vi "EINDE.vi"() -> ()   [LabVIEW 2018]
uses:
  Kleuren- en afstandsensor/FSM States.ctl
  FSM States Project TOTAAL.ctl
panel:
  out "Genoeg blokjes?":bool
  out "Initial State":T1=enum."MOVE DOWNWARDS"
  out "Tussentijd":i32
  out "Timer2":i32
  out "The End":bool
  in  "stop 3":bool
  in  "ON/OFF Grijper":bool
  in  "stop":bool
  in  "Aantal Witte blokjes":dbl
  in  "Aantal rode blokjes":dbl
  in  "Aantal Zwarte blokjes":dbl
  in  "LED aansturen":bool[](array[boolean])
  out "Current State":T1
  out "Motor":bool[](array[boolean])
  out "State to recover from":T1=enum."Stilstaan"
  in  "EMERGENCY":bool
  in  "Teller wit":dbl
  in  "Teller Rood":dbl
  in  "Teller zwart":dbl
  out "Wit":bool
  out "Zwart":bool
  out "Rood":bool
  in  "Kleurmaken":bool
  out "Kleuren veranderen":T2
  out "Analoge in":dbl[](array[numeric]) format="%0.2f"
  out "Afstand":bool
  # "INPUT"
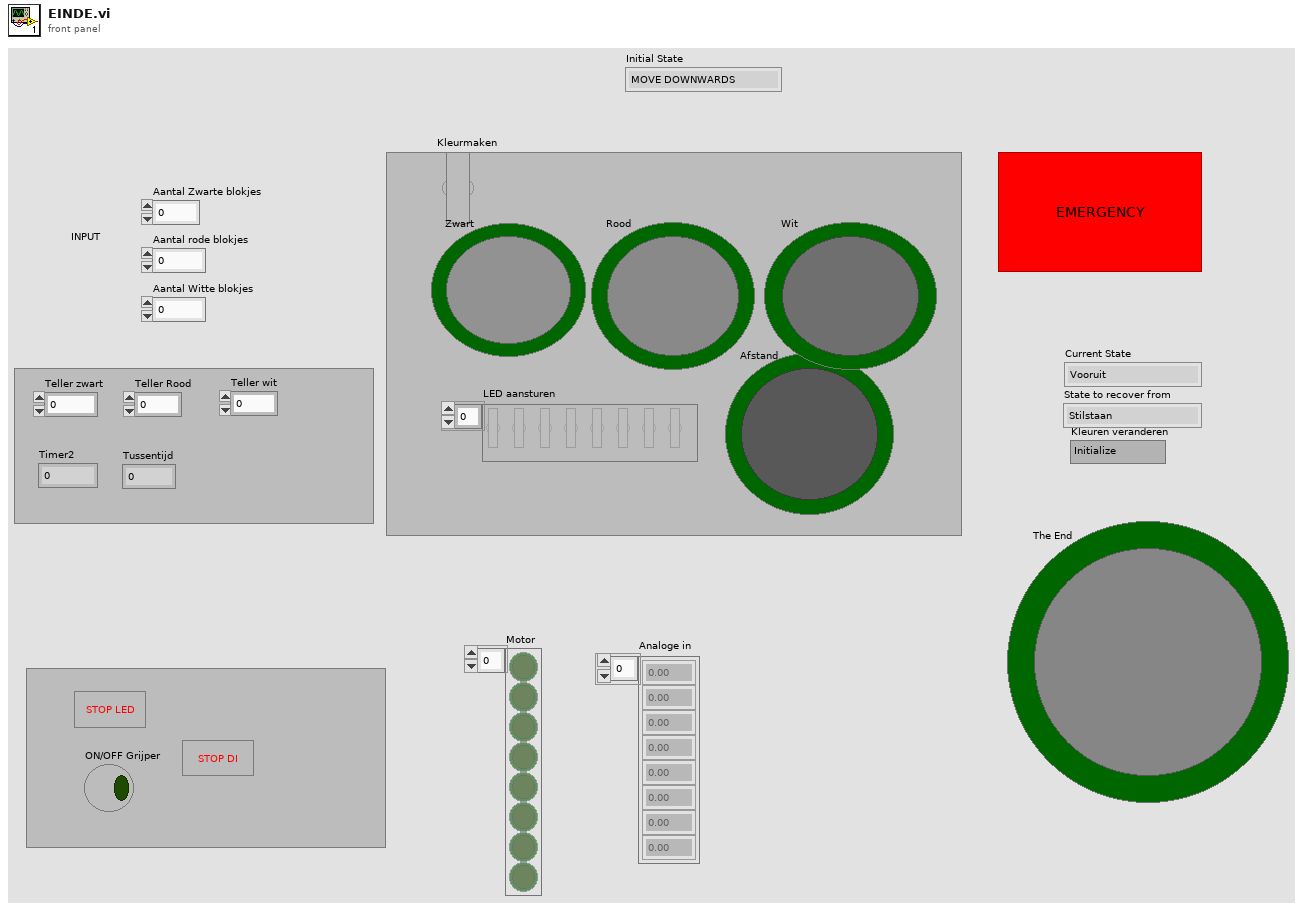
[diagram p1: front panel]
types:
  T1 = typedef "FSM States Project TOTAAL.ctl" = enum16{"Vooruit", "Achteruit", "Stilstaan", "EMERGENCY", "MOVE DOWNWARDS", "GRAB", "MOVE UPWARDS", "ROTATE", "DROP", "RETURN", "Stop "}
  T2 = typedef "FSM States.ctl" = enum16{"Initialize", "ROOD", "GROEN ", "Blauw "}
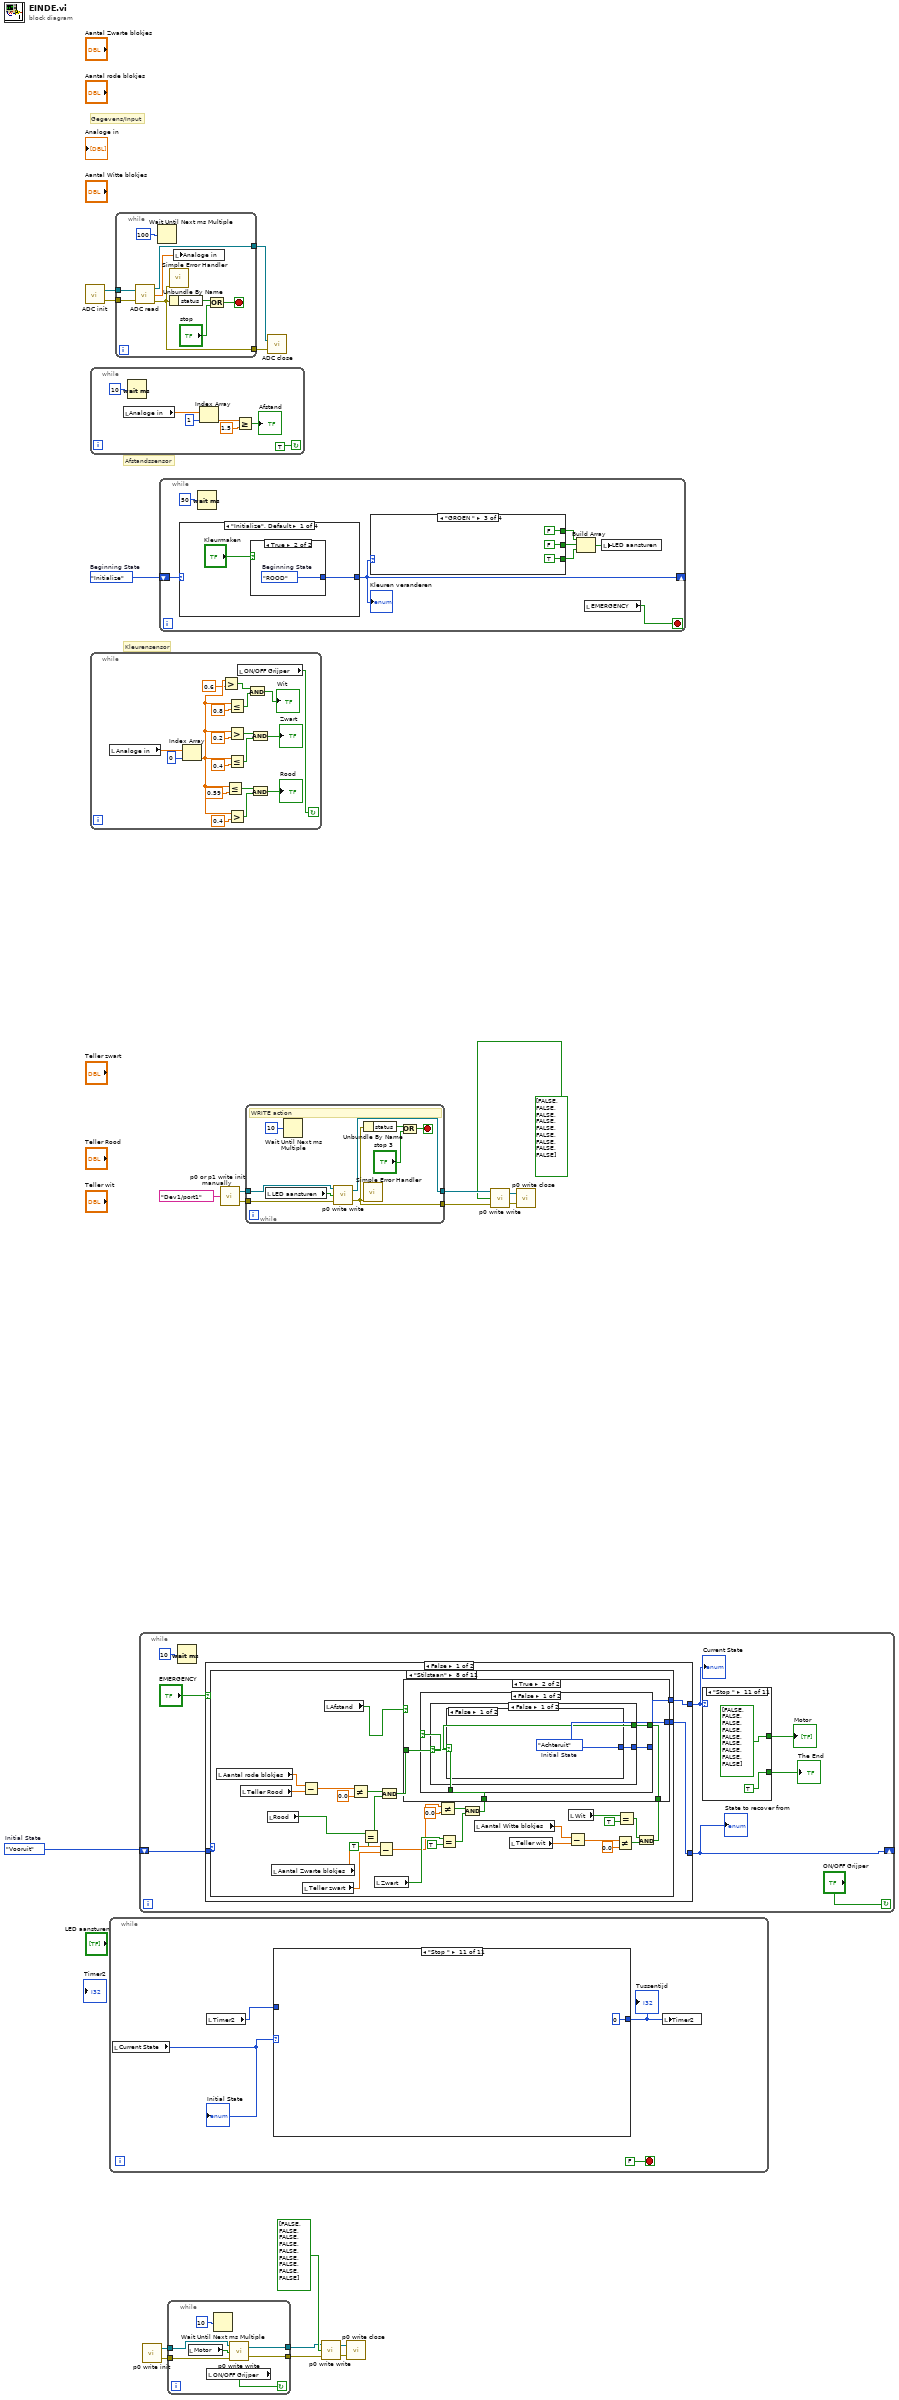
[diagram p0: block diagram]
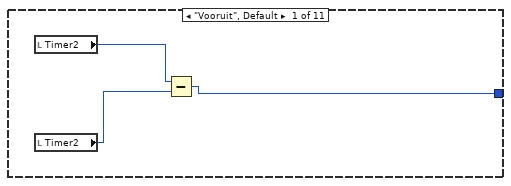
[diagram p2: hidden frame]
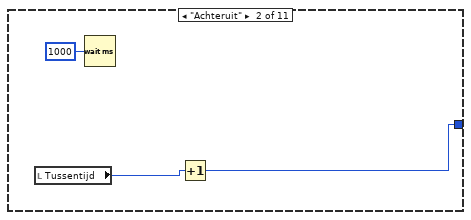
[diagram p3: hidden frame]
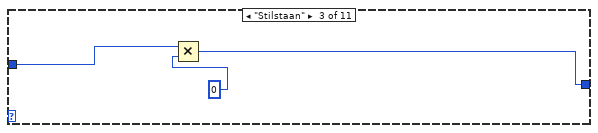
[diagram p4: hidden frame]
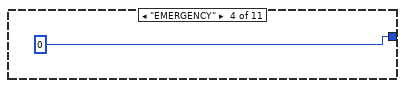
[diagram p5: hidden frame]
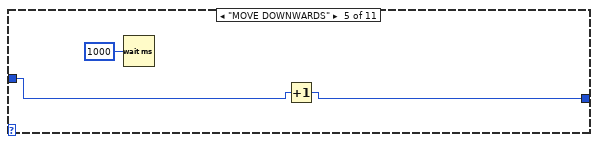
[diagram p6: hidden frame]
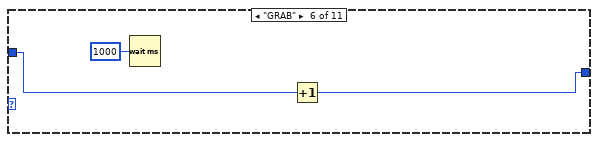
[diagram p7: hidden frame]
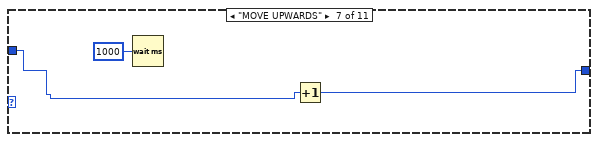
[diagram p8: hidden frame]
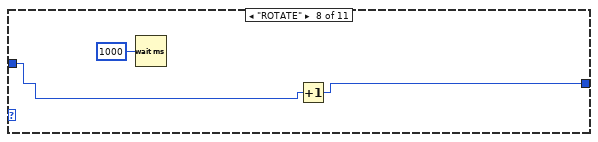
[diagram p9: hidden frame]
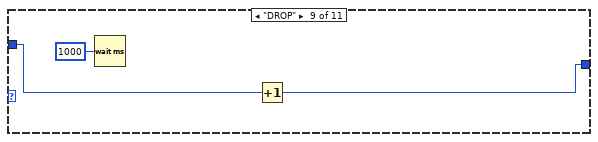
[diagram p10: hidden frame]
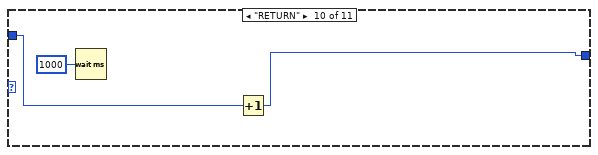
[diagram p11: hidden frame]
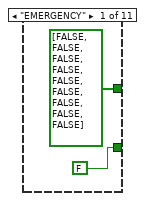
[diagram p12: hidden frame]
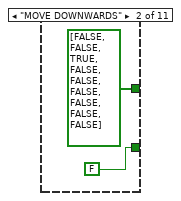
[diagram p13: hidden frame]
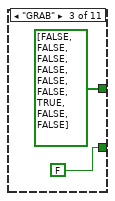
[diagram p14: hidden frame]
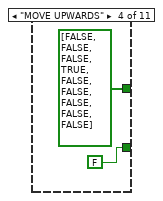
[diagram p15: hidden frame]
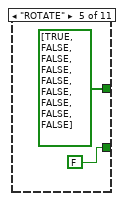
[diagram p16: hidden frame]
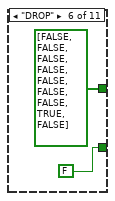
[diagram p17: hidden frame]
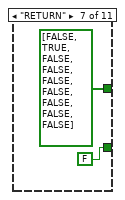
[diagram p18: hidden frame]
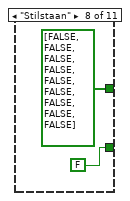
[diagram p19: hidden frame]
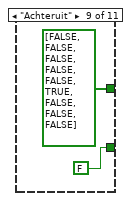
[diagram p20: hidden frame]
diagram:
  w1 = FSM_States_Project_TOTAAL."Vooruit"  # Initial State
  w17 = FSM_States."Initialize"  # Beginning State
  # "Gegevens/Input"
  # "Kleurensensor"
  # "Afstandssensor"
  n1 = call "ADC init.vi"() -> ("error out"=w20:errorcluster, "task out"=w21:refnum<k21>)
  n2 = while {
    stop <- TRUE continue-if-true
    n3 = local read "Analoge in"() -> (w22:dbl[])
    n4 = Wait (ms)(milliseconds to wait=u32 10) -> ()  [unwired: 1 out]
    n5 = Index Array(array=w22, index=1) -> (element=w26:dbl)
    n6 = Greater Or Equal?(x=w26, y=1.5) -> (x >= y?=→"Afstand":bool)
  }
  n7 = while {
    stop <- w34 continue-if-true
    n8 = local read "Analoge in"() -> (w46:dbl[])
    n9 = Index Array(array=w46, index=0) -> (element=w30:dbl)
    n10 = Greater?(x=w30, y=0.6) -> (0:w31:bool)
    n11 = Less Or Equal?(x=w30, y=0.59) -> (x <= y?=w36:bool)
    n12 = Less Or Equal?(x=w30, y=0.8) -> (x <= y?=w33:bool)
    n13 = Greater?(x=w30, y=0.2) -> (0:w42:bool)
    n14 = Less Or Equal?(x=w30, y=0.4) -> (x <= y?=w41:bool)
    n15 = Greater?(x=w30, y=0.4) -> (0:w35:bool)
    n16 = local read "ON/OFF Grijper"() -> (w34:bool)
    n17 = And(x=w31, y=w33) -> (x .and. y?=→"Wit":bool)
    n18 = And(x=w42, y=w41) -> (x .and. y?=→"Zwart":bool)
    n19 = And(x=w36, y=w35) -> (x .and. y?=→"Rood":bool)
  }
  n20 = while {
    stop <- FALSE stop-if-true
    n21 = local read "Current State"() -> (w48:T1)
    "Initial State" <- w48
    n22 = local read "Timer2"() -> (w50:i32)
    n23 = case shown="\"Stop \"" w48 {
      tunnel: w50 -> [_ _ w59 _ w63 w66 w69 w72 w75 w78 _]
      tunnel: [w54 w55 w58 0 ("Timer2") w62 w65 w68 w71 w74 w77 0 ("Timer2")] -> w49
      frame "Vooruit", Default {
        n24 = local read "Timer2"() -> (w52:i32)
        n25 = local read "Timer2"() -> (w53:i32)
        n26 = Subtract(x=w52, y=w53) -> (x-y=w54:i32)
      }
      frame "Achteruit" {
        n27 = local read "Tussentijd"() -> (w56:i32)
        n28 = Wait (ms)(milliseconds to wait=u32 1000) -> ()  [unwired: 1 out]
        n29 = Increment(x=w56) -> (x+1=w55:i32)
      }
      frame "Stilstaan" {
        n30 = Multiply(x=w59, y=0 ("Timer2")) -> (x*y=w58:i32)
      }
      frame "EMERGENCY" {
      }
      frame "MOVE DOWNWARDS" {
        n31 = Wait (ms)(milliseconds to wait=u32 1000) -> ()  [unwired: 1 out]
        n32 = Increment(x=w63) -> (x+1=w62:i32)
      }
      frame "GRAB" {
        n33 = Wait (ms)(milliseconds to wait=u32 1000) -> ()  [unwired: 1 out]
        n34 = Increment(x=w66) -> (x+1=w65:i32)
      }
      frame "MOVE UPWARDS" {
        n35 = Wait (ms)(milliseconds to wait=u32 1000) -> ()  [unwired: 1 out]
        n36 = Increment(x=w69) -> (x+1=w68:i32)
      }
      frame "ROTATE" {
        n37 = Wait (ms)(milliseconds to wait=u32 1000) -> ()  [unwired: 1 out]
        n38 = Increment(x=w72) -> (x+1=w71:i32)
      }
      frame "DROP" {
        n39 = Wait (ms)(milliseconds to wait=u32 1000) -> ()  [unwired: 1 out]
        n40 = Increment(x=w75) -> (x+1=w74:i32)
      }
      frame "RETURN" {
        n41 = Wait (ms)(milliseconds to wait=u32 1000) -> ()  [unwired: 1 out]
        n42 = Increment(x=w78) -> (x+1=w77:i32)
      }
      frame "Stop " {
      }
    }
    "Tussentijd" <- w49
    n43 = local write "Timer2"(w49) -> ()
  }
  n44 = while {
    tunnel: w21 -> [w89]
    tunnel: w20 -> [w88]
    tunnel: [w85] -> w19
    tunnel: [w87] -> w18
    stop <- w82 stop-if-true
    n45 = call "ADC read.vi"("task/channels in"=w89, "error in"=w88) -> ("task out"=w87:refnum<k21>, "analog in"=w81:dbl[], "error out"=w85:errorcluster)
    n46 = Wait Until Next ms Multiple(millisecond multiple=u32 100) -> ()  [unwired: 1 out]
    n47 = call <vilib>:"Simple Error Handler.vi"("error in (no error)"=w85) -> ()  [unwired: 4 in, 5 out]
    n48 = Unbundle By Name(w85) -> ("status"=w84:bool)
    n49 = local write "Analoge in"(w81) -> ()
    n50 = Or(x=w84, y="stop") -> (x .or. y?=w82:bool)
  }
  n51 = while {
    shift-right: [w93] -> _
    shift-left: w1 -> [w94]
    stop <- "ON/OFF Grijper" continue-if-true
    n52 = Wait (ms)(milliseconds to wait=u32 10) -> ()  [unwired: 1 out]
    n53 = case shown="False" "EMERGENCY" {
      tunnel: w94 -> [w122 _]
      tunnel: [w121 FSM_States_Project_TOTAAL."EMERGENCY" ("State to Recover from 2")] -> w92
      tunnel: [w120 w232] -> w93
      frame False {
        n54 = case shown="\"Stilstaan\"" w122 {
          tunnel: [w123 w124 w130 w136 w142 w148 w154 w188 w224 w227 w231] -> w121
          tunnel: [w123 w124 w130 w136 w142 w148 w154 w188 w224 w227 w231] -> w120
          frame "EMERGENCY" {
            n55 = local read "State to recover from"() -> (w123:T1)
          }
          frame "MOVE DOWNWARDS" {
            n56 = local read "Timer2"() -> (w127:i32)
            n57 = Greater Or Equal?(x=w127, y=8) -> (x >= y?=w125:bool)
            n58 = case shown="False" w125 {
              tunnel: [FSM_States_Project_TOTAAL."MOVE DOWNWARDS" FSM_States_Project_TOTAAL."GRAB"] -> w124
              frame False {
              }
              frame True {
              }
            }
          }
          frame "GRAB" {
            n59 = local read "Timer2"() -> (w132:i32)
            n60 = Greater Or Equal?(x=w132, y=10) -> (x >= y?=w133:bool)
            n61 = case shown="True" w133 {
              tunnel: [w134 w135] -> w130
              frame False {
                w134 = FSM_States_Project_TOTAAL."GRAB"  # Next State
              }
              frame True {
                w135 = FSM_States_Project_TOTAAL."MOVE UPWARDS"  # Next State
              }
            }
          }
          frame "MOVE UPWARDS" {
            n62 = local read "Timer2"() -> (w139:i32)
            n63 = Greater Or Equal?(x=w139, y=20) -> (x >= y?=w137:bool)
            n64 = case shown="True" w137 {
              tunnel: [w140 w141] -> w136
              frame False {
                w140 = FSM_States_Project_TOTAAL."MOVE UPWARDS"  # Next State
              }
              frame True {
                w141 = FSM_States_Project_TOTAAL."ROTATE"  # Next State
              }
            }
          }
          frame "ROTATE" {
            n65 = local read "Timer2"() -> (w145:i32)
            n66 = Greater Or Equal?(x=w145, y=23) -> (x >= y?=w143:bool)
            n67 = case shown="False" w143 {
              tunnel: [w146 w147] -> w142
              frame False {
                w146 = FSM_States_Project_TOTAAL."ROTATE"  # Next State
              }
              frame True {
                w147 = FSM_States_Project_TOTAAL."DROP"  # Next State
              }
            }
          }
          frame "DROP" {
            n68 = local read "Timer2"() -> (w151:i32)
            n69 = Greater Or Equal?(x=w151, y=25) -> (x >= y?=w149:bool)
            n70 = case shown="True" w149 {
              tunnel: [w152 w153] -> w148
              frame False {
                w152 = FSM_States_Project_TOTAAL."DROP"  # Next State
              }
              frame True {
                w153 = FSM_States_Project_TOTAAL."RETURN"  # Next State
              }
            }
          }
          frame "RETURN" {
            n71 = local read "Timer2"() -> (w156:i32)
            n72 = Greater Or Equal?(x=w156, y=28) -> (x >= y?=w157:bool)
            n73 = case shown="True" w157 {
              tunnel: [w158 w159] -> w154
              frame False {
                w158 = FSM_States_Project_TOTAAL."RETURN"  # Next State
              }
              frame True {
                w159 = FSM_States_Project_TOTAAL."Vooruit"  # Next State
              }
            }
          }
          frame "Stilstaan" {
            n74 = local read "Aantal rode blokjes"() -> (w178:dbl)
            n75 = local read "Teller Rood"() -> (w177:dbl)
            n76 = local read "Rood"() -> (w175:bool)
            n77 = local read "Aantal Zwarte blokjes"() -> (w185:dbl)
            n78 = Subtract(x=w178, y=w177) -> (x-y=w176:dbl)
            n79 = local read "Teller zwart"() -> (w187:dbl)
            n80 = local read "Afstand"() -> (w160:bool)
            n81 = Not Equal?(x=w176, y=0.0) -> (x != y?=w179:bool)
            n82 = Equal?(x=w175, y=TRUE) -> (x = y?=w174:bool)
            n83 = local read "Zwart"() -> (w186:bool)
            n84 = Subtract(x=w185, y=w187) -> (x-y=w184:dbl)
            n85 = And(x=w179, y=w174) -> (x .and. y?=w161:bool)
            n86 = Not Equal?(x=w184, y=0.0) -> (x != y?=w183:bool)
            n87 = Equal?(x=w186, y=TRUE) -> (x = y?=w182:bool)
            n88 = And(x=w183, y=w182) -> (x .and. y?=w171:bool)
            n89 = local read "Aantal Witte blokjes"() -> (w169:dbl)
            n90 = local read "Teller wit"() -> (w168:dbl)
            n91 = Subtract(x=w169, y=w168) -> (x-y=w167:dbl)
            n92 = local read "Wit"() -> (w170:bool)
            n93 = Not Equal?(x=w167, y=0.0) -> (x != y?=w165:bool)
            n94 = Equal?(x=w170, y=TRUE) -> (x = y?=w166:bool)
            n95 = And(x=w166, y=w165) -> (x .and. y?=w162:bool)
            n96 = case shown="True" w160 {
              tunnel: [w189 w193] -> w188
              tunnel: w161 -> [_ w192]
              tunnel: w171 -> [_ w191]
              tunnel: w162 -> [_ w190]
              frame False {
                w189 = FSM_States_Project_TOTAAL."Vooruit"  # Initial State
              }
              frame True {
                n97 = case shown="False" w192 {
                  tunnel: [w196 w208] -> w193
                  tunnel: w191 -> [w195 _]
                  tunnel: w190 -> [w194 _]
                  frame False {
                    n98 = case shown="False" w195 {
                      tunnel: [w197 w203] -> w196
                      tunnel: w194 -> [w198 _]
                      frame False {
                        n99 = case shown="False" w198 {
                          tunnel: [w199 w200] -> w197
                          frame False {
                            w199 = FSM_States_Project_TOTAAL."Achteruit"  # Initial State
                          }
                          frame True {
                            w200 = FSM_States_Project_TOTAAL."MOVE DOWNWARDS"  # Initial State
                            n100 = local read "Teller wit"() -> (w202:dbl)
                            n101 = Increment(x=w202) -> (x+1=w201:dbl)
                            n102 = local write "Teller wit"(w201) -> ()
                          }
                        }
                      }
                      frame True {
                        w203 = FSM_States_Project_TOTAAL."MOVE DOWNWARDS"  # Initial State
                        n103 = local read "Teller zwart"() -> (w205:dbl)
                        n104 = Increment(x=w205) -> (x+1=w204:dbl)
                        n105 = local write "Teller zwart"(w204) -> ()
                      }
                    }
                  }
                  frame True {
                    w208 = FSM_States_Project_TOTAAL."MOVE DOWNWARDS"  # Initial State
                    n106 = local read "Teller Rood"() -> (w207:dbl)
                    n107 = Increment(x=w207) -> (x+1=w206:dbl)
                    n108 = local write "Teller Rood"(w206) -> ()
                  }
                }
              }
            }
          }
          frame "Achteruit" {
            n109 = local read "Aantal Zwarte blokjes"() -> (w220:dbl)
            n110 = local read "Aantal rode blokjes"() -> (w217:dbl)
            n111 = local read "Teller zwart"() -> (w219:dbl)
            n112 = local read "Teller Rood"() -> (w216:dbl)
            n113 = local read "Aantal Witte blokjes"() -> (w214:dbl)
            n114 = local read "Teller wit"() -> (w213:dbl)
            n115 = Equal?(x=w220, y=w219) -> (x = y?=w218:bool)
            n116 = Equal?(x=w217, y=w216) -> (x = y?=w215:bool)
            n117 = local read "Tussentijd"() -> (w223:i32)
            n118 = Equal?(x=w214, y=w213) -> (x = y?=w212:bool)
            n119 = And(x=w218, y=w215) -> (x .and. y?=w221:bool)
            n120 = And(x=w221, y=w212) -> (x .and. y?=w209:bool)
            "Genoeg blokjes?" <- w209
            n121 = Equal?(x=w223, y=5) -> (x = y?=w210:bool)
            n122 = And(x=w209, y=w210) -> (x .and. y?=w211:bool)
            n123 = case shown="False" w211 {
              tunnel: [w225 w226] -> w224
              frame False {
                w225 = FSM_States_Project_TOTAAL."Achteruit"  # Initial State
              }
              frame True {
                w226 = FSM_States_Project_TOTAAL."Stop "  # Initial State
              }
            }
          }
          frame "Vooruit" {
            n124 = local read "Afstand"() -> (w228:bool)
            n125 = case shown="False" w228 {
              tunnel: [w229 w230] -> w227
              frame False {
                w229 = FSM_States_Project_TOTAAL."Vooruit"  # Initial State
              }
              frame True {
                w230 = FSM_States_Project_TOTAAL."Stilstaan"  # Initial State
              }
            }
          }
          frame "Stop " {
            w231 = FSM_States_Project_TOTAAL."Stop "  # Initial State
          }
        }
      }
      frame True {
        n126 = local read "State to recover from"() -> (w232:T1)
      }
    }
    "State to recover from" <- w93
    "Current State" <- w92
    n127 = case shown="\"Stop \"" w92 {
      tunnel: [bool[] [FALSE, FALSE, FALSE, FALSE, FALSE, FALSE, FALSE, FALSE, FALSE] ("digital out") bool[] [FALSE, FALSE, TRUE, FALSE, FALSE, FALSE, FALSE, FALSE, FALSE] ("digital out") bool[] [FALSE, FALSE, FALSE, FALSE, FALSE, FALSE, TRUE, FALSE, FALSE] ("digital out") bool[] [FALSE, FALSE, FALSE, TRUE, FALSE, FALSE, FALSE, FALSE, FALSE] ("digital out") bool[] [TRUE, FALSE, FALSE, FALSE, FALSE, FALSE, FALSE, FALSE, FALSE] ("digital out") bool[] [FALSE, FALSE, FALSE, FALSE, FALSE, FALSE, FALSE, TRUE, FALSE] ("digital out") bool[] [FALSE, TRUE, FALSE, FALSE, FALSE, FALSE, FALSE, FALSE, FALSE] ("digital out") bool[] [FALSE, FALSE, FALSE, FALSE, FALSE, FALSE, FALSE, FALSE, FALSE] ("digital out") bool[] [FALSE, FALSE, FALSE, FALSE, FALSE, TRUE, FALSE, FALSE, FALSE] ("digital out") bool[] [FALSE, FALSE, FALSE, FALSE, TRUE, FALSE, FALSE, FALSE, FALSE] ("digital out") bool[] [FALSE, FALSE, FALSE, FALSE, FALSE, FALSE, FALSE, FALSE, FALSE] ("digital out")] -> w90
      tunnel: [FALSE ("The End") FALSE ("The End") FALSE ("The End") FALSE ("The End") FALSE ("The End") FALSE ("The End") FALSE ("The End") FALSE ("The End") FALSE ("The End") FALSE ("The End") TRUE ("The End")] -> w91
      frame "EMERGENCY" {
      }
      frame "MOVE DOWNWARDS" {
      }
      frame "GRAB" {
      }
      frame "MOVE UPWARDS" {
      }
      frame "ROTATE" {
      }
      frame "DROP" {
      }
      frame "RETURN" {
      }
      frame "Stilstaan" {
      }
      frame "Achteruit" {
      }
      frame "Vooruit" {
      }
      frame "Stop " {
      }
    }
    "Motor" <- w90
    "The End" <- w91
  }
  n128 = call "p0 write init.vi"() -> ("error out"=w3:errorcluster, "task out"=w2:refnum<k21>)
  n129 = while {
    shift-right: [w235] -> _
    shift-left: w17 -> [w241]
    stop <- w234 stop-if-true
    n130 = case shown="\"Initialize\", Default" w241 {
      tunnel: [w255 w258 w259 w260] -> w235
      frame "Initialize", Default {
        n131 = case shown="True" "Kleurmaken" {
          tunnel: [w256 w257] -> w255
          frame False {
            w256 = FSM_States."Initialize"  # Beginning State
          }
          frame True {
            w257 = FSM_States."ROOD"  # Beginning State
          }
        }
      }
      frame "ROOD" {
        w258 = FSM_States."GROEN "  # Beginning State
      }
      frame "GROEN " {
        w259 = FSM_States."Blauw "  # Beginning State
      }
      frame "Blauw " {
        w260 = FSM_States."ROOD"  # Beginning State
      }
    }
    "Kleuren veranderen" <- w235
    n132 = Wait (ms)(milliseconds to wait=u32 50) -> ()  [unwired: 1 out]
    n133 = case shown="\"GROEN \"" w235 {
      tunnel: [FALSE FALSE FALSE TRUE] -> w238
      tunnel: [FALSE TRUE FALSE FALSE] -> w237
      tunnel: [FALSE FALSE TRUE FALSE] -> w236
      frame "Initialize", Default {
      }
      frame "ROOD" {
        # "Put the values of the outputs over here"
      }
      frame "GROEN " {
      }
      frame "Blauw " {
      }
    }
    n134 = Build Array(w238, w237, w236) -> (w239:bool[])
    n135 = local read "EMERGENCY"() -> (w234:bool)
    n136 = local write "LED aansturen"(w239) -> ()
  }
  n137 = while {
    tunnel: [w266] -> w5
    tunnel: [w265] -> w4
    tunnel: w3 -> [w263]
    tunnel: w2 -> [w264]
    stop <- w267 continue-if-true
    n138 = local read "Motor"() -> (w261:bool[])
    n139 = local read "ON/OFF Grijper"() -> (w267:bool)
    n140 = Wait Until Next ms Multiple(millisecond multiple=u32 10) -> ()  [unwired: 1 out]
    n141 = call "p0 write write.vi"("error in"=w263, "digital out"=w261, "task/channels in"=w264) -> ("error out"=w266:errorcluster, "task out"=w265:refnum<k21>)
  }
  n142 = call "p0 or p1 write init manually.vi"("Port"=tag "Dev1/port1") -> ("task out"=w11:refnum<k21>, "error out"=w10:errorcluster)
  n143 = while {
    tunnel: w11 -> [w276]
    tunnel: [w275] -> w16
    tunnel: w10 -> [w274]
    tunnel: [w270] -> w15
    stop <- w271 stop-if-true
    # "WRITE action"
    n144 = local read "LED aansturen"() -> (w268:bool[])
    n145 = Wait Until Next ms Multiple(millisecond multiple=u32 10) -> ()  [unwired: 1 out]
    n146 = call "p0 write write.vi"("error in"=w274, "digital out"=w268, "task/channels in"=w276) -> ("error out"=w270:errorcluster, "task out"=w275:refnum<k21>)
    n147 = Unbundle By Name(w270) -> ("status"=w269:bool)
    n148 = call <vilib>:"Simple Error Handler.vi"("error in (no error)"=w270) -> ()  [unwired: 4 in, 5 out]
    n149 = Or(x=w269, y="stop 3") -> (x .or. y?=w271:bool)
  }
  n150 = call "ADC close.vi"("error in"=w19, "task/channels in"=w18) -> ()
  n151 = call "p0 write write.vi"("error in"=w5, "digital out"=bool[] [FALSE, FALSE, FALSE, FALSE, FALSE, FALSE, FALSE, FALSE, FALSE], "task/channels in"=w4) -> ("error out"=w7:errorcluster, "task out"=w8:refnum<k21>)
  n152 = call "p0 write close.vi"("error in"=w7, "task/channels in"=w8) -> ()
  n153 = call "p0 write write.vi"("error in"=w15, "digital out"=bool[] [FALSE, FALSE, FALSE, FALSE, FALSE, FALSE, FALSE, FALSE, FALSE], "task/channels in"=w16) -> ("error out"=w13:errorcluster, "task out"=w14:refnum<k21>)
  n154 = call "p0 write close.vi"("error in"=w13, "task/channels in"=w14) -> ()
